vi "set_mc_scale_factor.vi"(8 "error in (no error)":errorcluster, 11 "TrajectoryMH100122AODRAPS in":refnum<class "TrajectoryMH100122AODRAPS.lvclass">) -> (0 "error out":errorcluster, 3 "TrajectoryMH100122AODRAPS out":refnum<class "TrajectoryMH100122AODRAPS.lvclass">)   [LabVIEW 2010, in "TrajectoryMH100122AODRAPS.lvclass"]
uses:
  TrajectoryMH100122AODRAPS.lvclass
  common/xcontrols/XImage/XImage/XImage.xctl
  TrajectoryMH100122AODRAPS.lvclass/TrajectoryMH100122AODRAPS.ctl
  class_data.vi
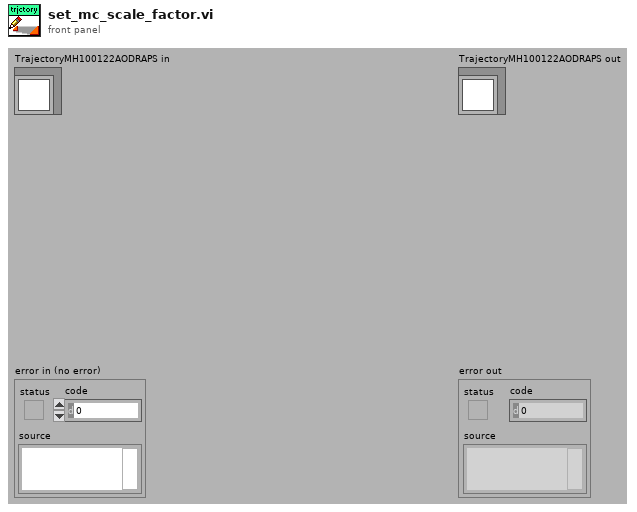
[diagram p1: front panel]
types:
  T1 = cluster{"Global Rectangle":i32[], "Contours":cluster{"Contour Type":u32, "ROI Type":u32, "Points":i32[]}[]}
  T2 = cluster{"Global Rectangle":i32[], "Contours":cluster{"Contour Type":u32, "ROI Type":u32, "Points":i32[]}[]}[]
  T3 = cluster{"Contour Type":u32, "ROI Type":u32, "Points":i32[]}[]
  T4 = typedef "IMAQ Rectangle" = cluster{"Left":i32, "Top":i32, "Right":i32, "Bottom":i32, "Rotation":dbl}
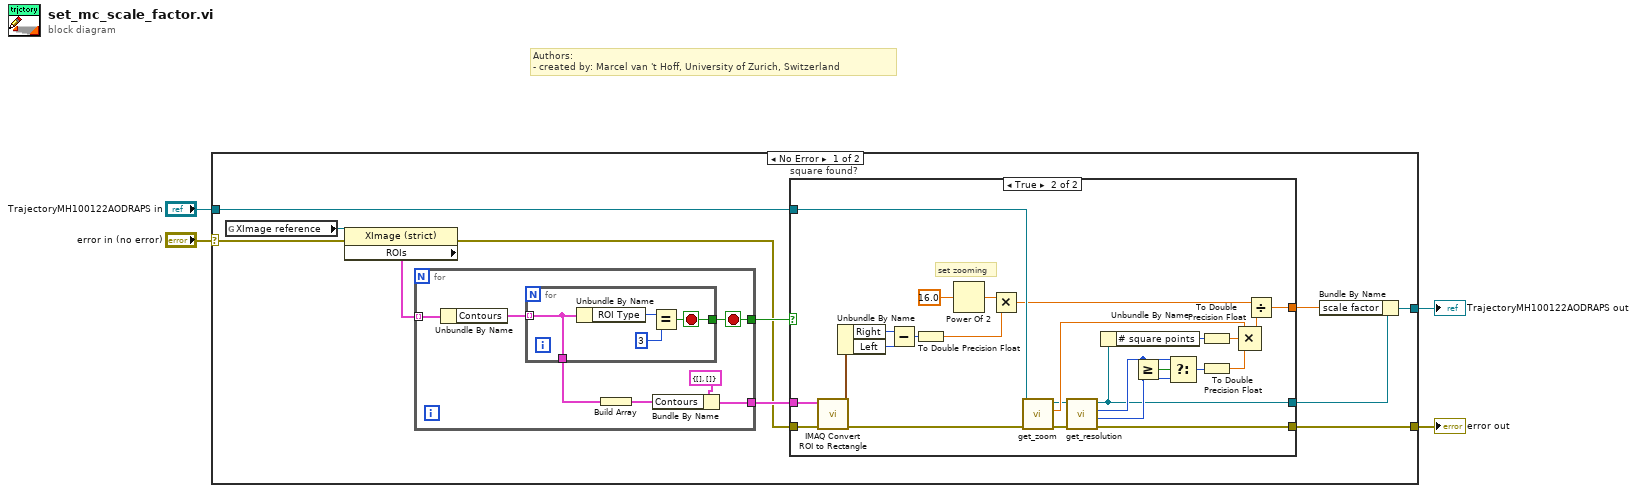
[diagram p0: block diagram]
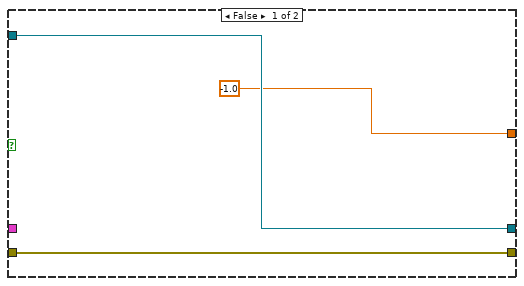
[diagram p2: hidden frame]
diagram:
  # "Authors: \n- created by: Marcel van 't Hoff, University of Zurich, Switzerland"
  n1 = case shown="No Error" "error in (no error)" {
    selector: "error in (no error)" -> [w14 w57]
    tunnel: [w9 w57] -> w3
    tunnel: [w5 w56] -> w1
    tunnel: "TrajectoryMH100122AODRAPS in" -> [w8 w56]
    frame No Error {
      n2 = global read "class_data.vi" "XImage reference"() -> (w13:refnum<vi>)
      n3 = property on="Property Node" class="XImage (strict)"(reference=w13, error in=w14) -> (error out=w10:errorcluster, "ROIs"=w15:T2)  [unwired: 1 out]
      n4 = for {
        tunnel: w15 -> [w50] mode=indexing
        tunnel: [w45] -> w11
        tunnel: [w51] -> w12
        stop <- w51 stop-if-true
        n5 = Unbundle By Name(w50) -> ("Contours"=w48:T3)
        n6 = for {
          tunnel: w48 -> [w52] mode=indexing
          tunnel: [w53] -> w51
          tunnel: [w52] -> w47
          stop <- w53 stop-if-true
          n7 = Unbundle By Name(w52) -> ("ROI Type"=w55:u32)
          n8 = Equal?(x=w55, y=u32 3) -> (x = y?=w53:bool)
        }
        n9 = Build Array(w47) -> (w46:T3)
        n10 = Bundle By Name(cluster=T1 {"Global Rectangle"=[], "Contours"=[]} ("ROI"), "Contours"=w46) -> (w45:T1)
      }
      n11 = case "square found?" shown="True" w12 {
        tunnel: w11 -> [_ w43]
        tunnel: w10 -> [w18 w42]
        tunnel: [w18 w22] -> w9
        tunnel: w8 -> [w17 w26]
        tunnel: [w17 w25] -> w6
        tunnel: [-1.0 w35] -> w7
        frame False {
        }
        frame True {
          # "set zooming"
          n12 = call "IMAQ Convert ROI to Rectangle"("error in (no error)"=w42, "ROI Descriptor"=w43) -> ("error out"=w23:errorcluster, "Rectangle"=w44:T4)  [unwired: 7 in]
          n13 = Unbundle By Name(w44) -> ("Right"=w41:i32, "Left"=w40:i32)
          n14 = Subtract(x=w41, y=w40) -> (x-y=w39:i32)
          n15 = To Double Precision Float(number=w39) -> (double precision float=w33:dbl)
          n16 = Power Of 2(x=16.0) -> (2^x=w34:dbl)
          n17 = Multiply(x=w34, y=w33) -> (x*y=w19:dbl)
          n18 = call-dynamic "get_zoom.vi"("error in (no error)"=w23, "TrajectoryMH100122AODRAPS in"=w26) -> ("error out"=w24:errorcluster, "zoom"=w28:dbl, "TrajectoryMH100122AODRAPS out"=w27:refnum<class "TrajectoryMH100122AODRAPS.lvclass">)  [unwired: 7 in]
          n19 = call-dynamic "get_resolution.vi"("error in (no error)"=w24, "TrajectoryMH100122AODRAPS in"=w27) -> ("error out"=w22:errorcluster, "y resolution"=w32:u32, "x resolution"=w31:u32, "TrajectoryMH100122AODRAPS out"=w25:refnum<class "TrajectoryMH100122AODRAPS.lvclass">)  [unwired: 6 in]
          n20 = Unbundle By Name(w25) -> ("# square points"=w38:i32)
          n21 = Greater Or Equal?(x=w31, y=w32) -> (x >= y?=w30:bool)
          n22 = Select(t=w31, s=w30, f=w32) -> (s? t:f=w29:u32)
          n23 = To Double Precision Float(number=w38) -> (double precision float=w20:dbl)
          n24 = To Double Precision Float(number=w29) -> (double precision float=w21:dbl)
          n25 = Compound Arithmetic op=MULTIPLY(w28, w20, w21) -> (w36:dbl)
          n26 = Divide(x=w19, y=w36) -> (x/y=w35:dbl)
        }
      }
      n27 = Bundle By Name(cluster=w6, "scale factor"=w7) -> (w5:refnum<class "TrajectoryMH100122AODRAPS.lvclass">)
    }
    frame Error {
    }
  }
  "error out" <- w3
  "TrajectoryMH100122AODRAPS out" <- w1
